vi "Command Get Tote Into Robot.vi"(2 "Input Robot System Funtions":T1, 3 "Cmd Parameter 1":dbl, 4 "Cmd Parameter 2":dbl, 5 "Startup":bool) -> (0 "Output Robot System Functions":T1, 1 "Completed":bool)   [LabVIEW 2014]
uses:
  Subsystems VIs/Robot Commands.ctl
  Command Execution State.ctl
  Global Variables/Sensor Data (Edited).vi
  Global Variables/Settings.vi
panel:
  out "Driver Switch 2":bool
  out "PID Tracking":cluster{"Goal Wheel Position":dbl, dbl}(graph)={"Goal Wheel Position"=0.0, -90.17571233858979}
  # "Sample robot\ncontrol output.\nReplace with \nactual teleop \ncontrol signal \nstructure."
  # "Field Centric"
  # "Field Centric"
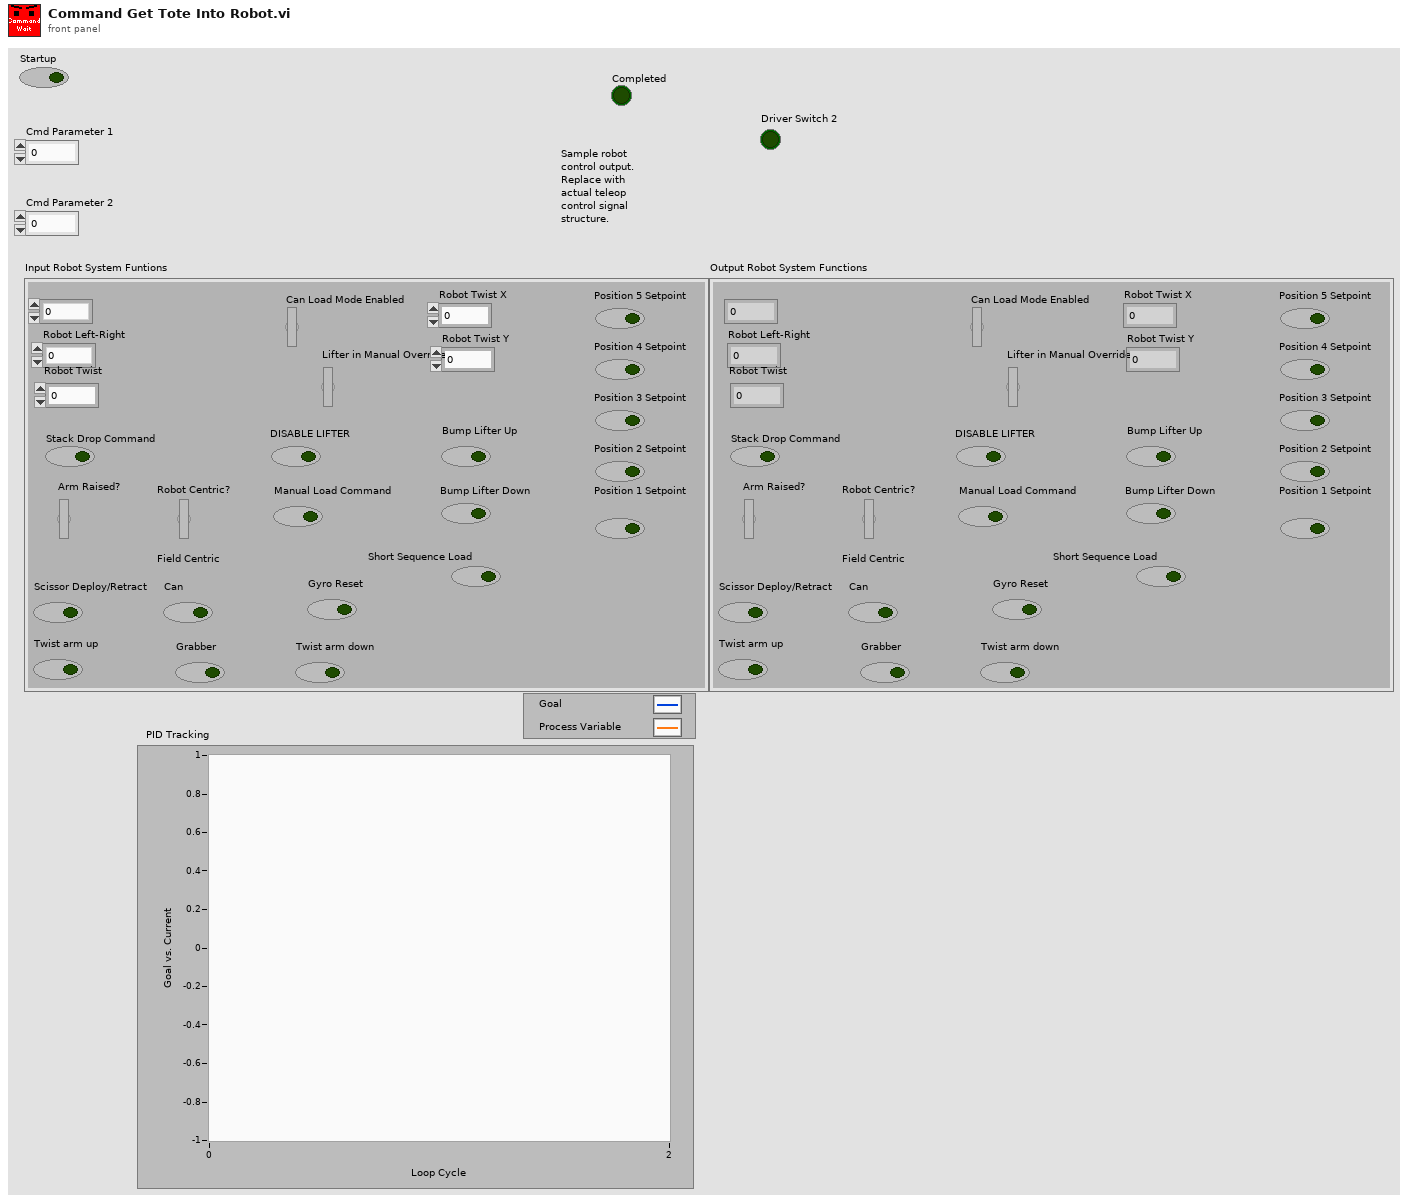
[diagram p1: front panel]
types:
  T1 = typedef "Robot Commands.ctl" = cluster{"Robot Forward-Reverse":dbl, "Robot Left-Right":dbl, "Robot Twist":dbl, "Can Load Mode Enabled":bool, "Lifter in Manual Override?":bool, "Stack Drop Command":bool, "Arm Raised?":bool, "DISABLE LIFTER":bool, "Position 1 Setpoint":bool, "Position 2 Setpoint":bool, "Position 3 Setpoint":bool, "Position 4 Setpoint":bool, "Position 5 Setpoint":bool, "Bump Lifter Down":bool, "Bump Lifter Up":bool, "Manual Load Command":bool, "Robot Centric?":bool, "Scissor Deploy/Retract":bool, "Grabber":bool, "Can":bool, "Twist arm up":bool, "Gyro Reset":bool, "Twist arm down":bool, "Short Sequence Load":bool, "Robot Twist X":dbl, "Robot Twist Y":dbl}
  T2 = typedef "Command Execution State.ctl" = enum16{"Initialize", "Execute", "Finish"}
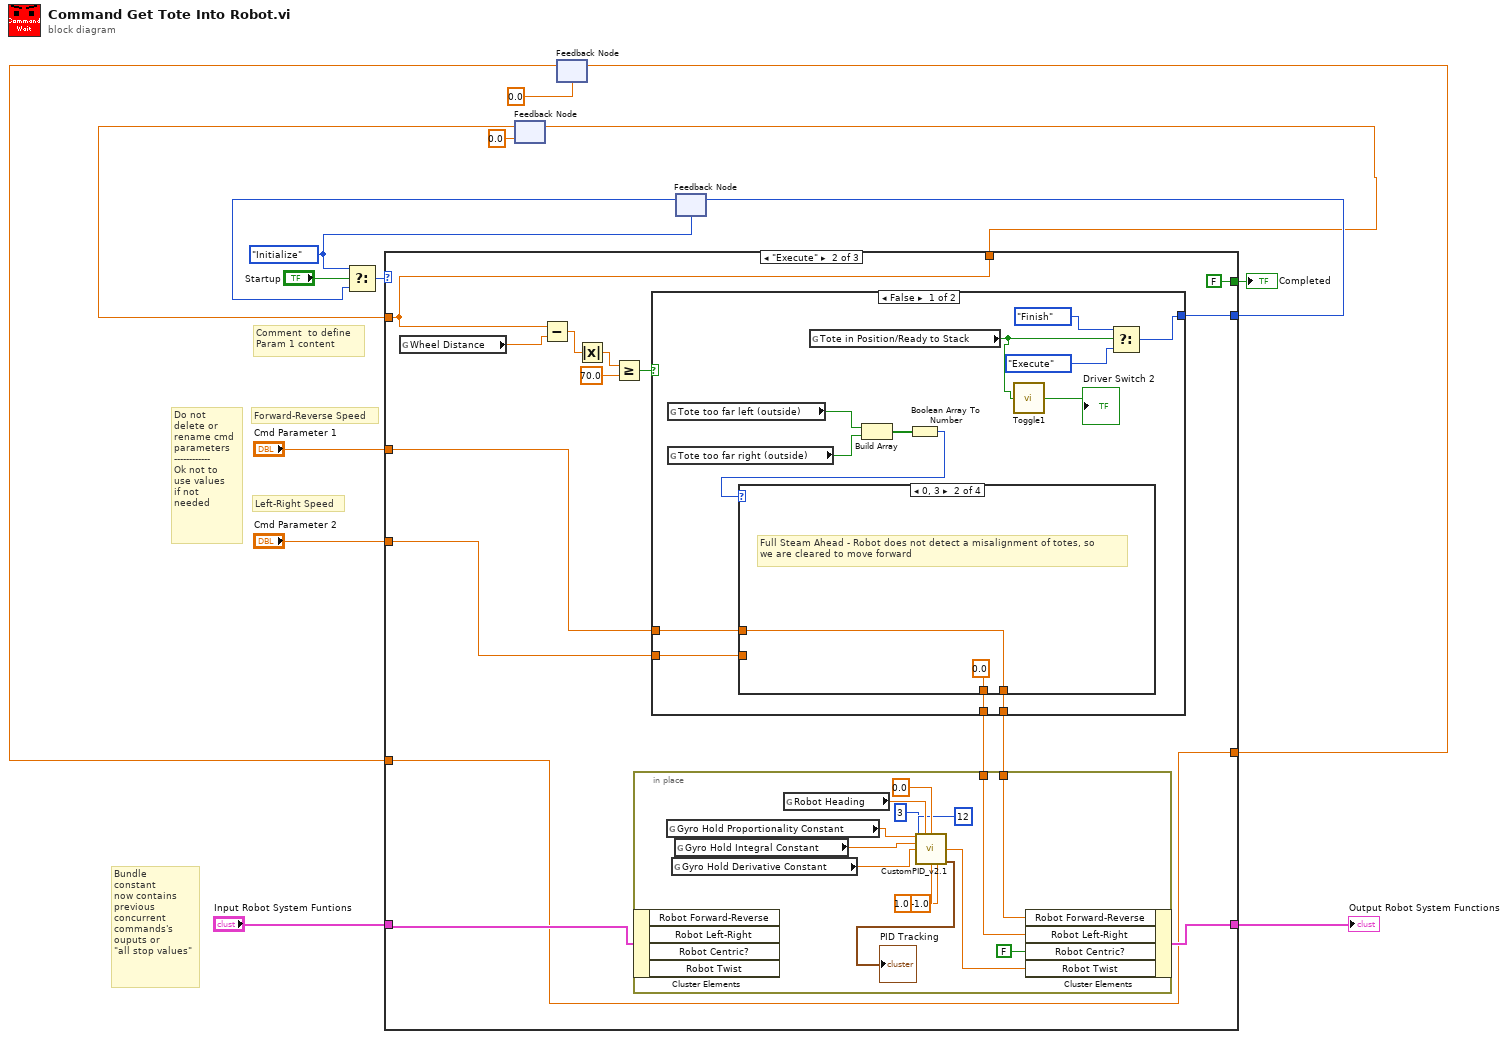
[diagram p0: block diagram]
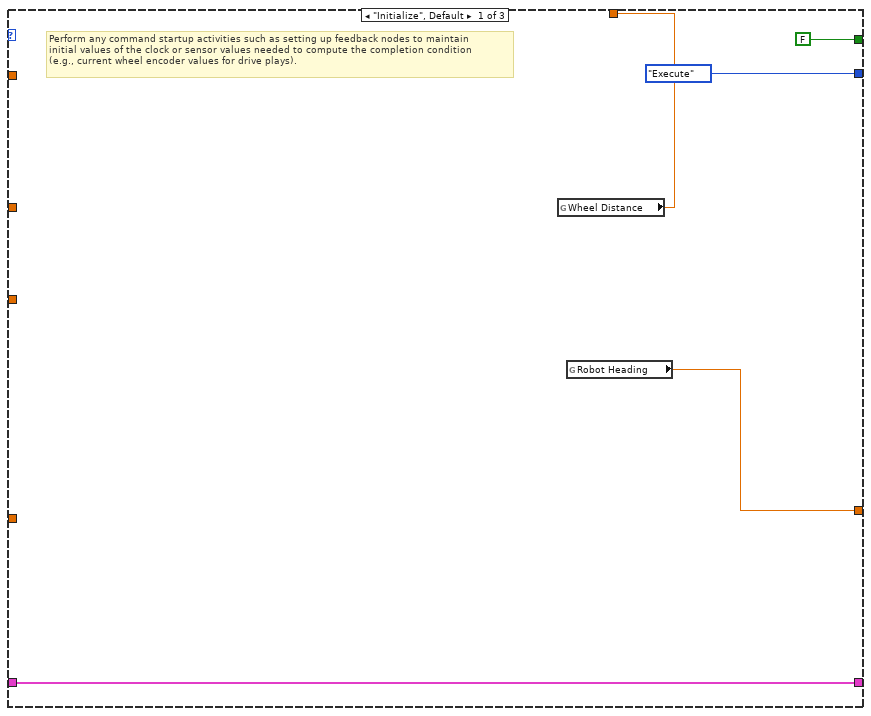
[diagram p2: hidden frame]
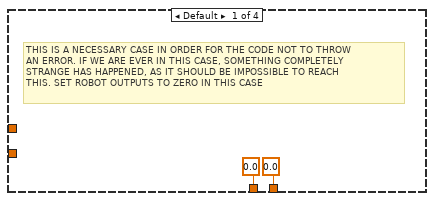
[diagram p3: hidden frame]
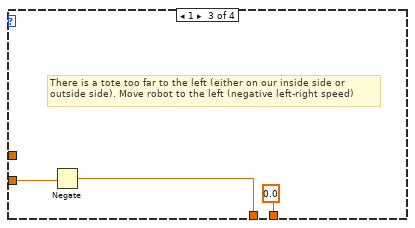
[diagram p4: hidden frame]
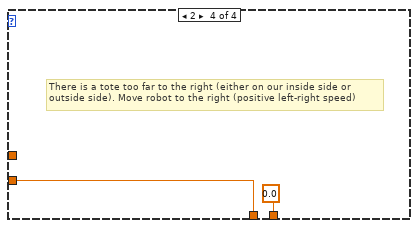
[diagram p5: hidden frame]
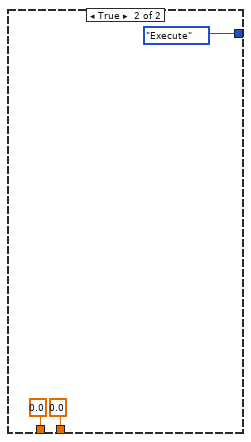
[diagram p6: hidden frame]
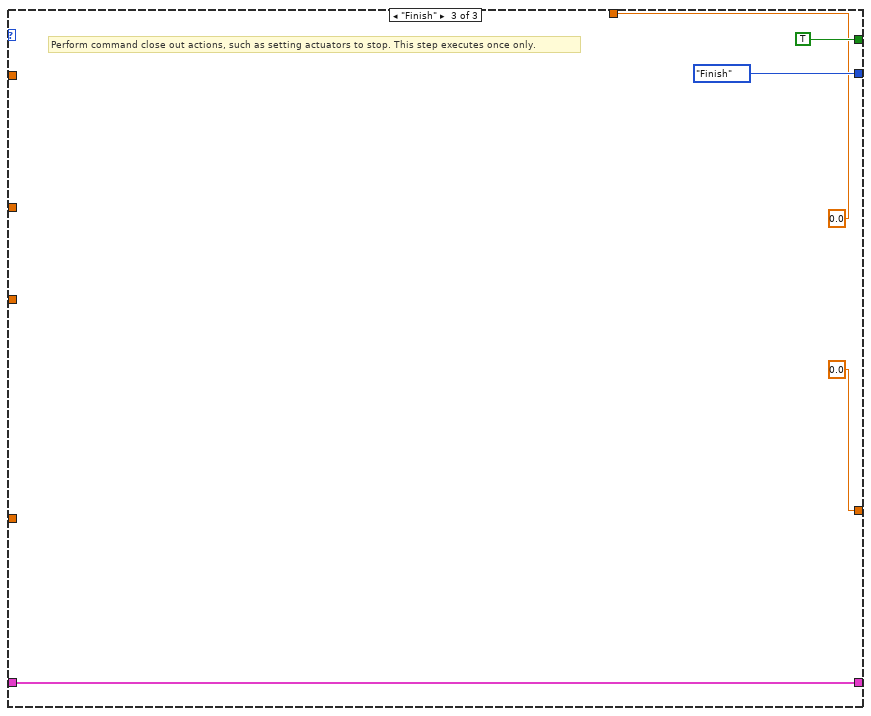
[diagram p7: hidden frame]
diagram:
  w11 = Command_Execution_State."Initialize" ("Play State")
  # "Forward-Reverse Speed"
  # "Bundle \nconstant\nnow contains\nprevious \nconcurrent\ncommands's\nouputs or\n\"all stop values\""
  # "Do not \ndelete or\nrename cmd\nparameters\n------------\nOk not to \nuse values\nif not \nneeded"
  # "Left-Right Speed"
  # "Comment  to define\nParam 1 content"
  n1 = feedback #1(0.0 ("Wheel Distance")) -> (w6:dbl)
  n2 = feedback #2(0.0 ("Wheel Distance")) -> (w3:dbl)
  n3 = feedback #3(w11) -> (w12:T2)
  n4 = Select(t=w11, s="Startup", f=w12) -> (s? t:f=w16:T2)
  n5 = case shown="\"Execute\"" w16 {
    tunnel: [FALSE FALSE TRUE] -> w14
    tunnel: [Command_Execution_State."Execute" ("Play State") w22 Command_Execution_State."Finish" ("f")] -> w13
    tunnel: "Cmd Parameter 1" -> [_ w26 _]
    tunnel: "Cmd Parameter 2" -> [_ w25 _]
    tunnel: [w19 w35 w76] -> w7
    tunnel: "Input Robot System Funtions" -> [w19 w36 w76]
    tunnel: [w18 w30 0.0 ("Wheel Distance")] -> w1
    tunnel: w6 -> [_ w30 _]
    tunnel: [w17 w28 0.0 ("Wheel Distance")] -> w4
    tunnel: w3 -> [_ w28 _]
    frame "Initialize", Default {
      # "Perform any command startup activities such as setting up feedback nodes to maintain \ninitial values of the clock or sensor values needed to compute the completion condition\n(e.g., current wheel encoder values for drive plays)."
      n6 = global read "Sensor Data (Edited).vi" "Wheel Distance"() -> (w18:dbl)
      n7 = global read "Sensor Data (Edited).vi" "Robot Heading"() -> (w17:dbl)
    }
    frame "Execute" {
      n8 = global read "Sensor Data (Edited).vi" "Wheel Distance"() -> (w34:dbl)
      n9 = Subtract(x=w30, y=w34) -> (x-y=w33:dbl)
      n10 = Absolute Value(x=w33) -> (abs(x)=w32:dbl)
      n11 = Greater Or Equal?(x=w32, y=70.0) -> (x >= y?=w27:bool)
      n12 = case shown="False" w27 {
        tunnel: w26 -> [w47 _]
        tunnel: w25 -> [w46 _]
        tunnel: [w45 0.0 ("Cmd Parameter 1")] -> w24
        tunnel: [w44 0.0 ("Cmd Parameter 2")] -> w23
        tunnel: [w41 Command_Execution_State."Execute" ("f")] -> w22
        frame False {
          n13 = global read "Sensor Data (Edited).vi" "Tote too far left (outside)"() -> (w37:bool)
          n14 = global read "Sensor Data (Edited).vi" "Tote too far right (outside)"() -> (w38:bool)
          n15 = global read "Sensor Data (Edited).vi" "Tote in Position/Ready to Stack"() -> (w40:bool)
          n16 = Build Array(w37, w38) -> (w49:bool[])
          n17 = Boolean Array To Number(Boolean array=w49) -> (number=w48:u32)
          n18 = case shown="0, 3" w48 {
            tunnel: w47 -> [_ w53 _ _]
            tunnel: w46 -> [_ _ w56 w58]
            tunnel: [0.0 ("Cmd Parameter 1") w53 0.0 ("Cmd Parameter 1") 0.0 ("Cmd Parameter 1")] -> w45
            tunnel: [0.0 ("Cmd Parameter 2") 0.0 ("Cmd Parameter 2") w55 w58] -> w44
            frame Default {
              # "THIS IS A NECESSARY CASE IN ORDER FOR THE CODE NOT TO THROW\nAN ERROR. IF WE ARE EVER IN THIS CASE, SOMETHING COMPLETELY \nSTRANGE HAS HAPPENED, AS IT SHOULD BE IMPOSSIBLE TO REACH \nTHIS. SET ROBOT OUTPUTS TO ZERO IN THIS CASE"
            }
            frame 0, 3 {
              # "Full Steam Ahead - Robot does not detect a misalignment of totes, so\nwe are cleared to move forward"
            }
            frame 1 {
              # "There is a tote too far to the left (either on our inside side or\noutside side). Move robot to the left (negative left-right speed)"
              n19 = Negate(x=w56) -> (-x=w55:dbl)
            }
            frame 2 {
              # "There is a tote too far to the right (either on our inside side or\noutside side). Move robot to the right (positive left-right speed)"
            }
          }
          n20 = call "Toggle1.vi"("Boolean"=w40) -> ("Driver Switch 2"=→"Driver Switch 2":bool)
          n21 = Select(t=Command_Execution_State."Finish" ("f"), s=w40, f=Command_Execution_State."Execute") -> (s? t:f=w41:T2)
        }
        frame True {
        }
      }
      n22 = in-place {
        in-place-border: w24 -> [w63]
        in-place-border: w23 -> [w62]
        n23 = in-place-cluster #4(w36) -> ()  [unwired: 4 out]
        n24 = global read "Settings.vi" "Gyro Hold Proportionality Constant"() -> (w67:dbl)
        n25 = global read "Settings.vi" "Gyro Hold Derivative Constant"() -> (w65:dbl)
        n26 = global read "Settings.vi" "Gyro Hold Integral Constant"() -> (w66:dbl)
        n27 = global read "Sensor Data (Edited).vi" "Robot Heading"() -> (w73:dbl)
        n28 = call "CustomPID_v2.1.vi"("Kp"=w67, "Process Variable"=w73, "Goal"=0.0 ("Setpoint"), "Ki"=w66, "Kd"=w65, "N-Diff"=3, "N-Int"=12, "Max Ouput"=1.0, "Min Output"=-1.0) -> ("Command"=w74:dbl, "PID Tracking"=→"PID Tracking":cluster{"Goal Wheel Position":dbl, dbl})  [unwired: 4 in, 1 out]
        n29 = in-place-cluster #4("Robot Forward-Reverse"=w63, "Robot Left-Right"=w62, "Robot Centric?"=FALSE, "Robot Twist"=w74) -> (w35:T1)
      }
    }
    frame "Finish" {
      # "Perform command close out actions, such as setting actuators to stop. This step executes once only."
    }
  }
  "Completed" <- w14
  "Output Robot System Functions" <- w7
  n30 = feedback-in #1(w1) -> ()
  n31 = feedback-in #2(w4) -> ()
  n32 = feedback-in #3(w13) -> ()
